vi "SSC Digital Write Static.vi"(0 "Digital SSC in":T1[](array[typedef]), 5 "State":T2 items=["0"=0, "1"=1, "X"=5], 11 "error in":errorcluster) -> (4 "Digital SSC out":T1[](array[typedef]), 15 "error out":errorcluster)   [LabVIEW 2020]
doc: "Writes a static state to all specified pin(s) and pin group(s). The selected pins remain in the specified state until the next pattern burst or call to this VI. If there are uncommitted changes to levels or the termination mode, this VI commits the changes to the pins.\n\nThis VI does not change the selected pin function. If you write a static state to a pin that does not have the Digital function selected, the new static state is stored by the digital pattern instrument, and affects the state of the pin the next time you change the selected function to Digital."
uses:
  <instrlib>/niDigital/niDigital.llb/niDigital Write Static Pin State.ctl
  SSC Digital.ctl
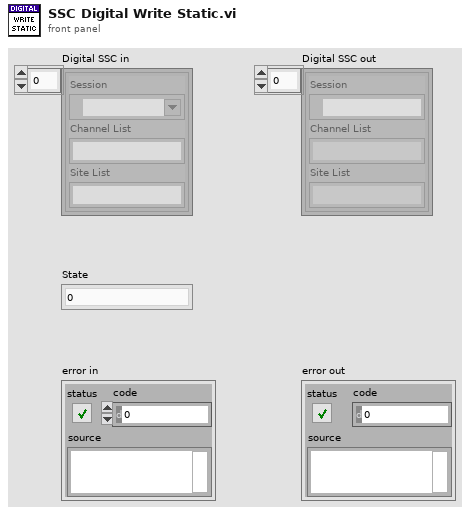
[diagram p1: front panel]
types:
  T1 = typedef "SSC Digital.ctl" = cluster{"Session":refnum<k15>, "Channel List":string, "Site List":string}
  T2 = typedef "niDigital Write Static Pin State.ctl" = u8
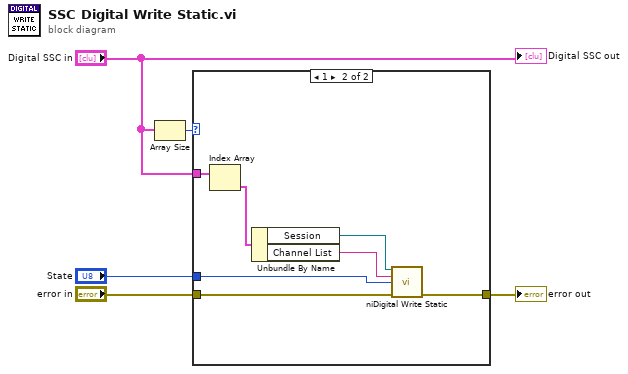
[diagram p0: block diagram]
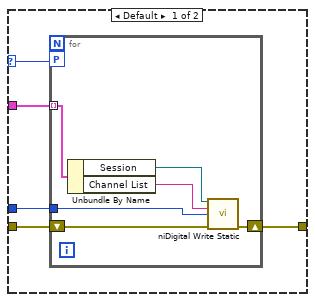
[diagram p2: hidden frame]
diagram:
  n1 = Array Size(array="Digital SSC in") -> (size(s)=w2:i32)
  n2 = case shown="1" w2 {
    selector: w2 -> [w7 _]
    tunnel: "State" -> [w10 w23]
    tunnel: "error in" -> [w9 w22]
    tunnel: [w8 w21] -> w3
    tunnel: "Digital SSC in" -> [w6 w20]
    frame Default {
      n3 = for {
        workers-P: w7 -> [_]
        tunnel: w10 -> [w14]
        tunnel: w6 -> [w13] mode=indexing
        shift-right: [w15] -> w8
        shift-left: w9 -> [w16]
        n4 = Unbundle By Name(w13) -> ("Session"=w11:refnum<k15>, "Channel List"=w12:string)
        n5 = call <instrlib>:"niDigital Write Static.vi"("instrument handle"=w11, "channel list"=w12, "state"=w14, "error in"=w16) -> ("error out"=w15:errorcluster)  [unwired: 10 in, 1 out]
      }
    }
    frame 1 {
      n6 = Index Array(array=w20) -> (element=w17:T1)  [unwired: 1 in]
      n7 = Unbundle By Name(w17) -> ("Session"=w18:refnum<k15>, "Channel List"=w19:string)
      n8 = call <instrlib>:"niDigital Write Static.vi"("instrument handle"=w18, "channel list"=w19, "state"=w23, "error in"=w22) -> ("error out"=w21:errorcluster)  [unwired: 10 in, 1 out]
    }
  }
  "error out" <- w3
  "Digital SSC out" <- "Digital SSC in"
